vi "Set All Pin Low.vi"(8 "error in (no error)":errorcluster, 11 "PEU in":refnum<class "PEU.lvclass">) -> (0 "error out":errorcluster, 3 "PEU out":refnum<class "PEU.lvclass">)   [LabVIEW 2020, in "PEU.lvlib" / "PEU.lvclass"]
uses:
  PEU.lvclass
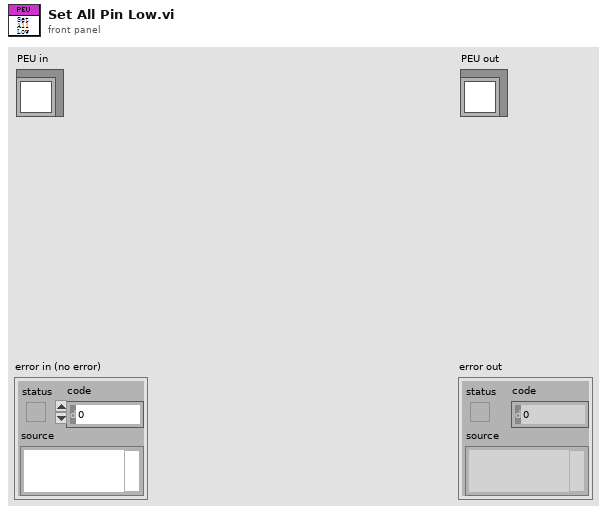
[diagram p1: front panel]
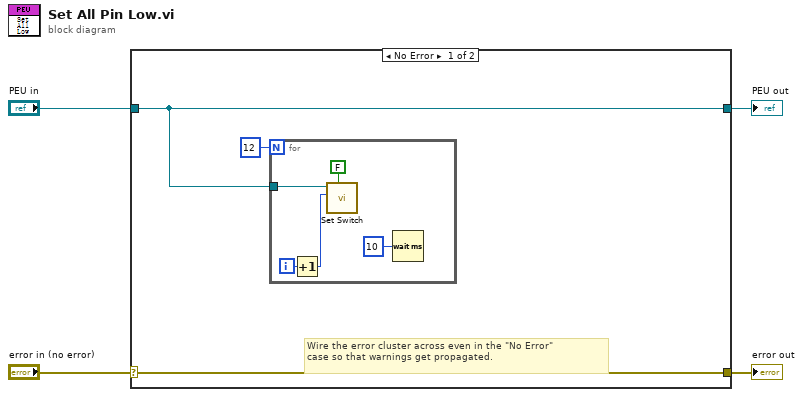
[diagram p0: block diagram]
diagram:
  n1 = case shown="No Error" "error in (no error)" {
    selector: "error in (no error)" -> [w7 w14]
    tunnel: [w7 w14] -> w3
    tunnel: [w5 w13] -> w1
    tunnel: "PEU in" -> [w5 w13]
    frame No Error {
      # "Wire the error cluster across even in the \"No Error\"\ncase so that warnings get propagated."
      n2 = for {
        N: 12 -> [_]
        tunnel: w5 -> [w9]
        i -> [w12]
        n3 = Increment(x=w12) -> (x+1=w11:i32)
        n4 = call "Set Switch.vi"("ON/OFF"=FALSE, "Pin"=w11, "PEU in"=w9) -> ()  [unwired: 7 in, 2 out]
        n5 = Wait (ms)(milliseconds to wait=u32 10) -> ()  [unwired: 1 out]
      }
    }
    frame Error {
    }
  }
  "error out" <- w3
  "PEU out" <- w1
